vi "Filter Options.vi"(10 "Text":string, 11 "All Options":string[](array[string])) -> (3 "Filtered Names":string[](array[string]))   [LabVIEW 2020, in "AutoComplete.lvlib"]
uses:
  AutoComplete.lvlib
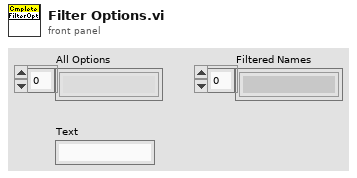
[diagram p1: front panel]
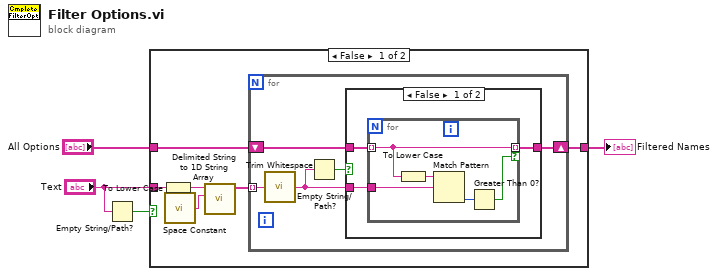
[diagram p0: block diagram]
diagram:
  n1 = Empty String/Path?(string/path="Text") -> (empty?=w1:bool)
  n2 = case shown="False" w1 {
    tunnel: [w10 w25] -> w4
    tunnel: "All Options" -> [w9 w25]
    tunnel: "Text" -> [w8 _]
    frame False {
      n3 = To Lower Case(string=w8) -> (all lower case string=w7:string)
      n4 = call <vilib>:"Space Constant.vi"() -> ("String"=w6:string)
      n5 = call <vilib>:"Delimited String to 1D String Array.vi"("delimiter"=w6, "delimited string"=w7) -> ("string array"=w5:string[])  [unwired: 9 in]
      n6 = for {
        shift-right: [w15] -> w10
        shift-left: w9 -> [w14]
        tunnel: w5 -> [w13] mode=indexing
        n7 = call <vilib>:"Trim Whitespace.vi"("string"=w13) -> ("trimmed string"=w12:string)  [unwired: 1 in]
        n8 = Empty String/Path?(string/path=w12) -> (empty?=w11:bool)
        n9 = case shown="False" w11 {
          tunnel: [w18 w24] -> w15
          tunnel: w14 -> [w17 w24]
          tunnel: w12 -> [w16 _]
          frame False {
            n10 = for {
              tunnel: w16 -> [w21]
              tunnel: [w20] -> w18 mode=indexing if=w22
              tunnel: w17 -> [w20] mode=indexing
              n11 = To Lower Case(string=w20) -> (all lower case string=w19:string)
              n12 = Match Pattern(string=w19, regular expression=w21) -> (offset past match=w23:i32)  [unwired: 1 in, 3 out]
              n13 = Greater Than 0?(x=w23) -> (x > 0?=w22:bool)
            }
          }
          frame True {
          }
        }
      }
    }
    frame True {
    }
  }
  "Filtered Names" <- w4
